vi "测试应用程序2.vi"() -> ()   [LabVIEW 2022 SP3]
doc: "本VI是为《我和LabVIEW》一书编写的示例。\n关于本书的介绍请参考网页：\nhttp://ruanqizhen.spaces.live.com/blog/cns!5852D4F797C53FB6!4310.entry"
panel:
  out "数据":dbl
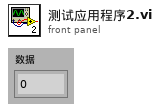
[diagram p1: front panel]
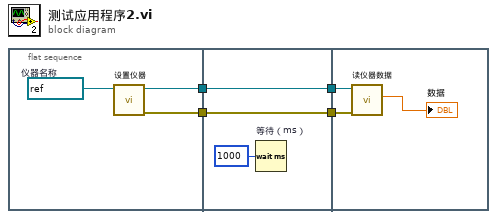
[diagram p0: block diagram]
diagram:
  n1 = flat-sequence {
    tunnel: [w6] -> w3
    tunnel: [w5] -> w1
    tunnel: [w9] -> w4
    tunnel: w3 -> [w9]
    tunnel: [w8] -> w2
    tunnel: w1 -> [w8]
    tunnel: w4 -> [w12]
    tunnel: w2 -> [w11]
    frame #0 {
      w7 = refnum<visa-resource-name> "XX仪"  # 仪器名称
      n2 = call "设置仪器.vi"("VISA资源名称"=w7) -> ("error out"=w5:errorcluster, "仪器句柄"=w6:refnum<visa-resource-name>)  [unwired: 1 in, 8 out]
    }
    frame #1 {
      n3 = Wait (ms) "等待（ms）"(milliseconds to wait=u32 1000 ("等待时间（毫秒）")) -> ()  [unwired: 1 out]
    }
    frame #2 {
      n4 = call "读仪器数据.vi"("error in (no error)"=w11, "仪器句柄"=w12) -> ("数据"=→"数据":dbl)  [unwired: 9 out]
    }
  }
